vi "cs-scanning_ssxy.vi"() -> ()   [LabVIEW 2017]
uses:
  controls/boolean_info.ctl
  controls/z-axis-params_ssxy.ctl
  <vilib>/rvi/Emulation/niFpgaGetClockAttributes.vi
  <vilib>/rvi/Emulation/niFpgaSctlEmulationGetInTimedLoop.vi
  <vilib>/rvi/Emulation/niFpgaEmulationReportErrorSimple.vi
  <vilib>/rvi/Emulation/niFpgaProcessEmulError.vi
  <vilib>/rvi/eio/common/nirviEmuTemplateMethod_errors.vi
  <vilib>/rvi/Emulation/niFpgaCriticalErrorInLSC.vi
  <vilib>/rvi/Emulation/niFpgaEmulationIsFPGAContextNoSignature.vi
  <vilib>/rvi/DataTransferAndStorage/Container/Common/niFpgaContainerGetUniqueNameForEmu.vi
  <vilib>/rvi/Memory/Memory_Emulation/niFpgaMemoryEmulationCacheClearOnFirstRun.vi
  <vilib>/rvi/Memory/Memory_Emulation/nirvimemoryEmulationManagerCache_MakeExclusive.vi
  <vilib>/rvi/Memory/Memory_Emulation/niFpgaMemoryEmulationValidateCache.vi
  <vilib>/rvi/Memory/Memory_Emulation/nirvimemoryEmulationManagerCache_InsertValue.vi
  <vilib>/Utility/error.llb/Clear Errors.vi
  <vilib>/rvi/Memory/Memory_Emulation/nirvimemoryEmulationManagerCache_ReleaseExclusive.vi
  <vilib>/rvi/Memory/Memory_Emulation/nirvimemoryEmulationManagerCache_GetValue.vi
  <vilib>/rvi/Memory/Memory_Emulation/nirvimemoryEmulationManagerCache_SetValue.vi
  <vilib>/eio/EIONode/EIONode.xnode
  <vilib>/rvi/DataTransferAndStorage/Container/XNode/niFpgaContainer.xnode
  <vilib>/rvi/DataTransferAndStorage/Register/Emulation/niFpgaRegisterEmulation.vi
  FPGA-data-logging.lvlib
  libimaging-cs.lvlib
panel:
  out "xy(k)":fxp<+/-,17,6>[](array[numeric])
  out "ref-data":fxp<+/-,16,5>[](array[numeric])
  out "u_y saturated":bool
  out "u_x saturated":bool
  in  "Ki-xy 2":sgl=0.001 format="%#_13g"
  in  "xy-bound 2":sgl
  out "scaning finished 2":bool
  out "scaning finished":bool
  out "Stopped 2":bool
  in  "z_axis_params":T1={"TOL"=0.29998779296875, "ramp_rate"=-5e-06, "z_u_max"=5.0, "setpoint"=0.0, "Ki"=0.001007080078125, "Z_error_threshold"=0.0, "Z_settled_samples_threshold "=0, "z_UP"=1.5, "zup_N"=5000} {"Z_error_threshold" format="%#_13g"; "ramp_rate" format="%#_4g"; "TOL" format="%#_13g"}
  in  "Kiz_down":sgl format="%#_13g"
  in  "max_Z_settle_samples":i16
  in  "step_down_frac":fxp<+,8,1>
  in  "collect all":bool
  out "iter":i32
  out "entity-index":i16
  in  "TsTicks":u32=1600
  out "number-settled-samples-Z":i16
  out "State":i8
  out "boolean \nindicators":T2
  out "z-u(k)":fxp<+/-,16,5>
  in  "ABORT":bool
  out "read fifo timeout":bool
  in  "numEntities":i16
  in  "init Z up":fxp<+/-,16,5>
  in  "trigger-0":bool
  out "number-settled-samples-y":i16
  out "number-settled-samples-x":i16
  in  "xy-error-threshold":sgl format="%#_13g"
  in  "settled-samples\nthreshold":i16
  in  "initial case":i8
  # "- If collect all = fasle and collect move = false,\nwe only collect measurement data.\n- If collect all = false, and collect move = true,\nwe collect measurement and move data.\n- If collect all = true, we collect everything."
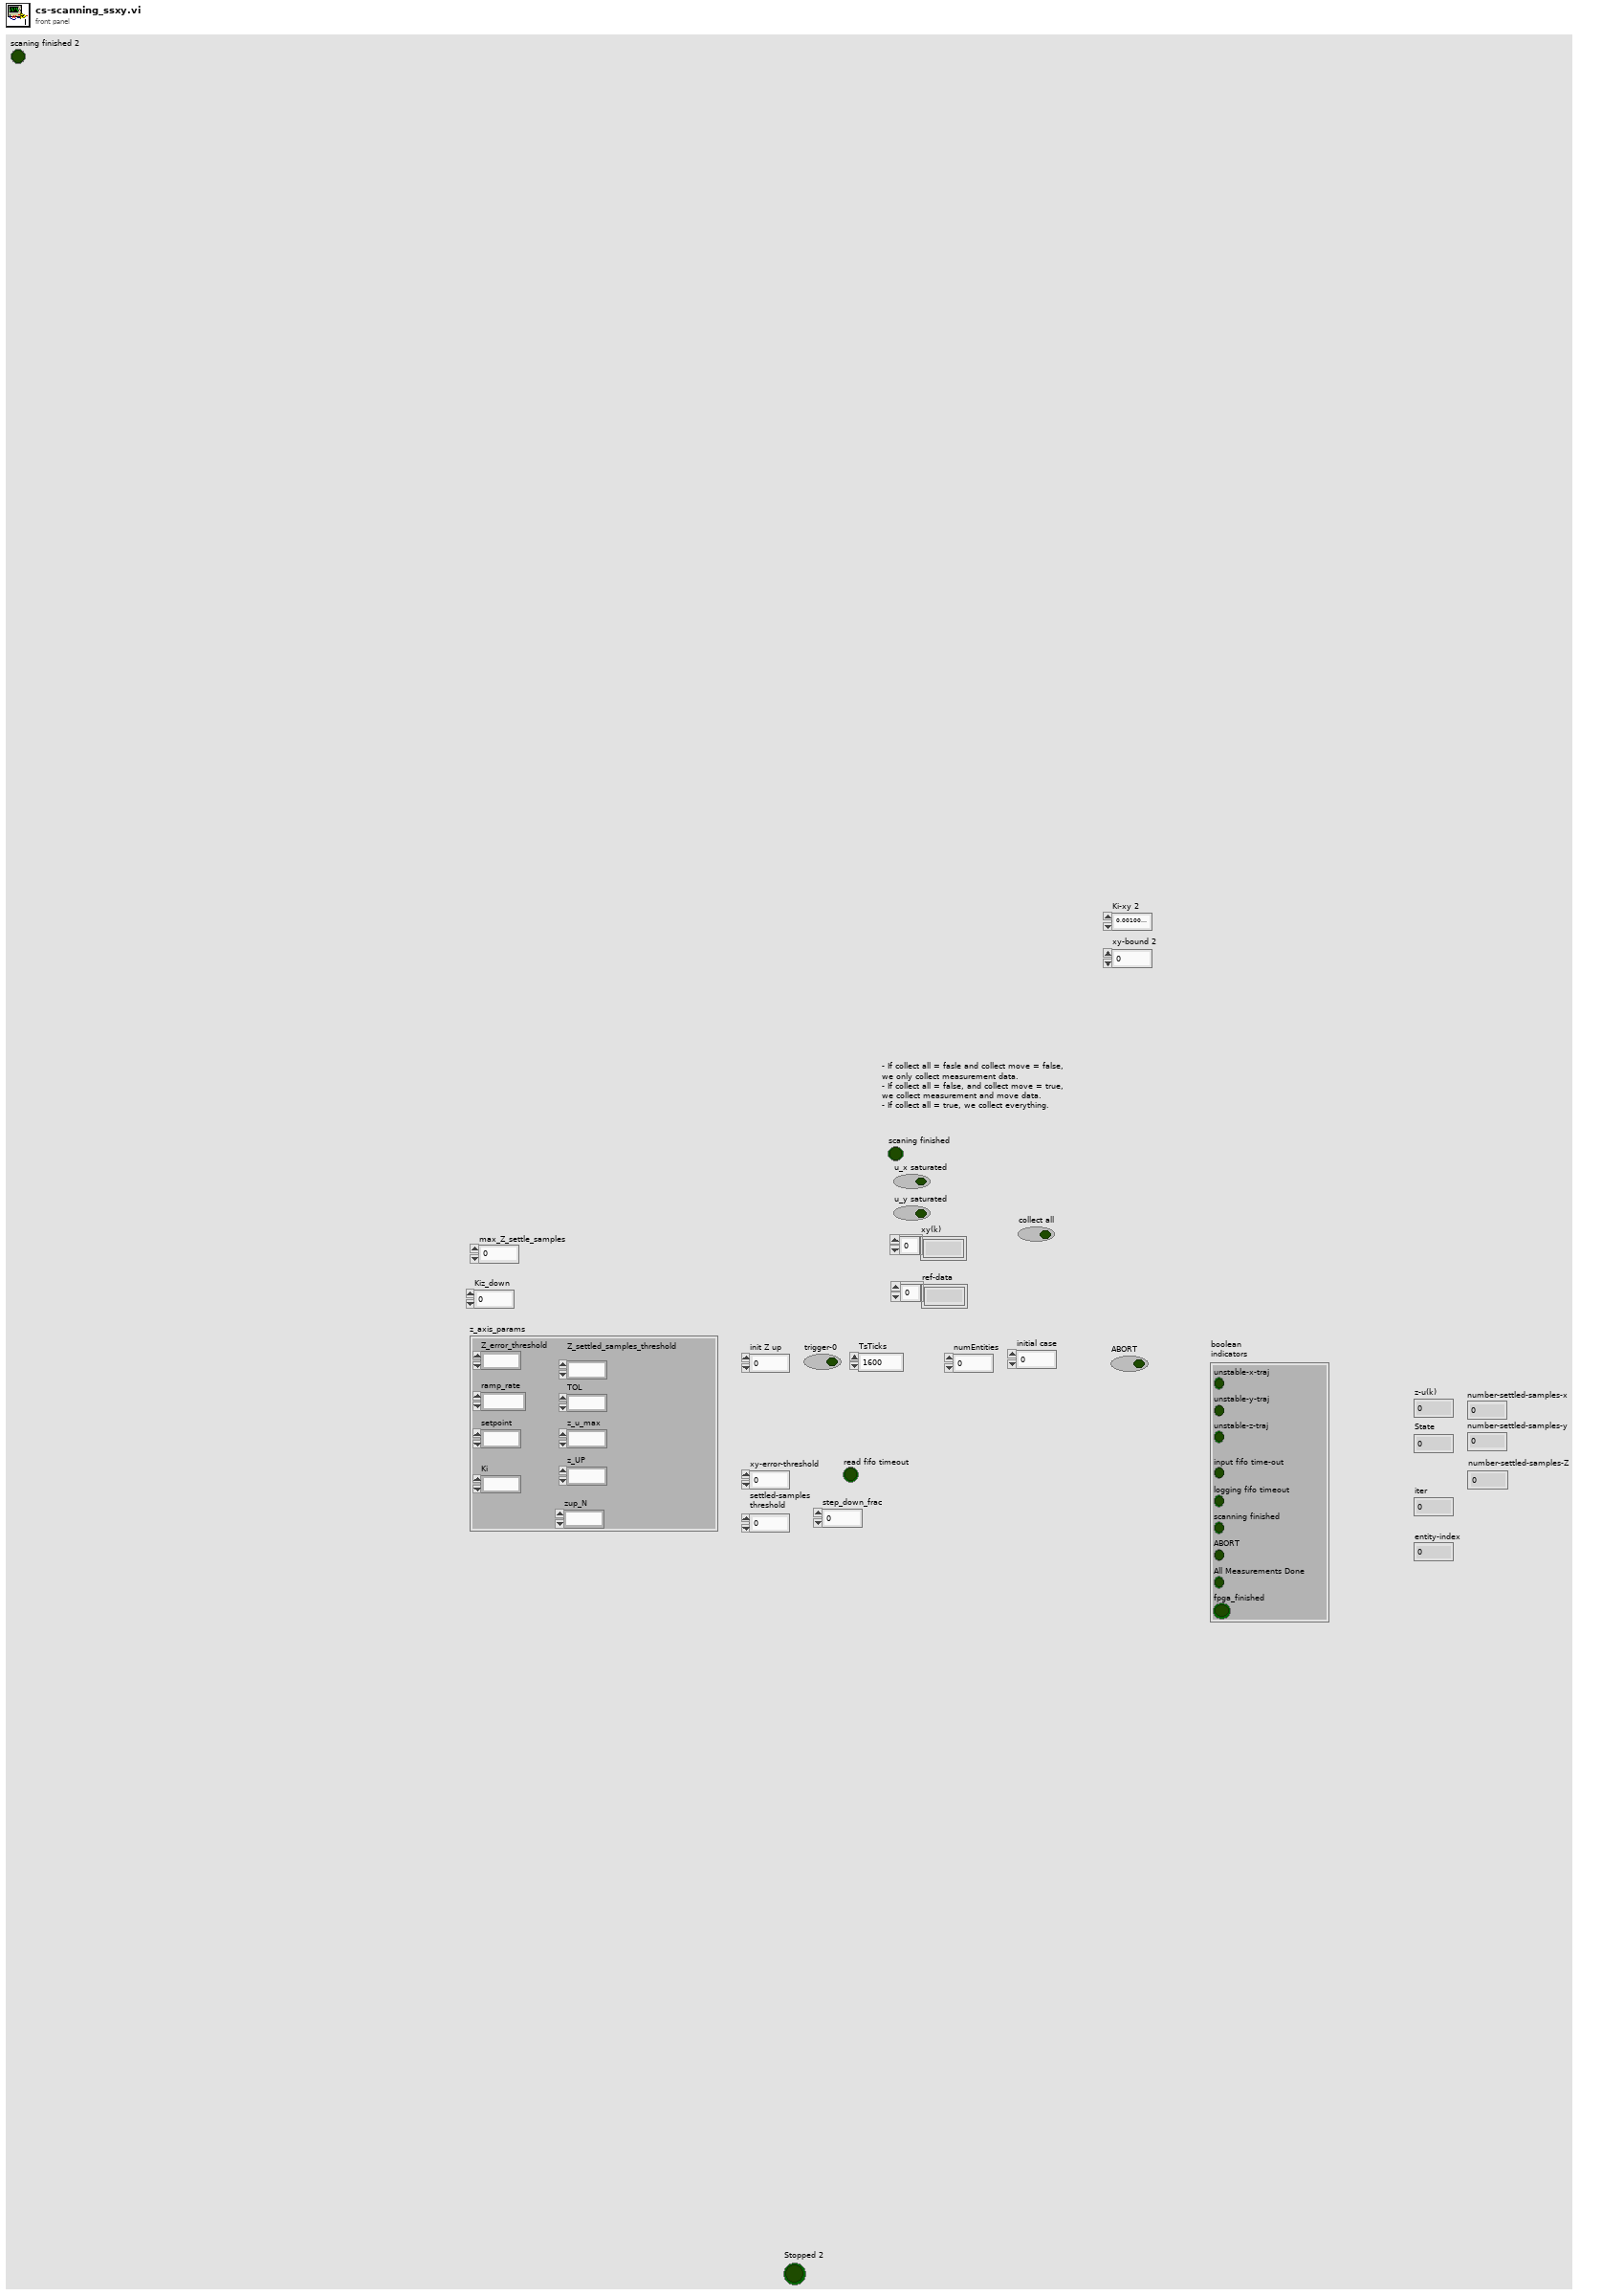
[diagram p1: front panel]
types:
  T1 = typedef "z-axis-params_ssxy.ctl" = cluster{"TOL":fxp<+/-,16,2>, "ramp_rate":sgl, "z_u_max":fxp<+/-,16,5>, "setpoint":fxp<+/-,16,5>, "Ki":fxp<+,16,1>, "Z_error_threshold":fxp<+/-,16,5>, "Z_settled_samples_threshold ":i16, "z_UP":fxp<+/-,16,5>, "zup_N":i16}
  T2 = typedef "boolean_info.ctl" = cluster{"unstable-z-traj":bool, "input fifo time-out":bool, "logging fifo timeout":bool, "scanning finished":bool, "unstable-x-traj":bool, "unstable-y-traj":bool, "ABORT":bool, "All Measurements Done":bool, "fpga_finished":bool}
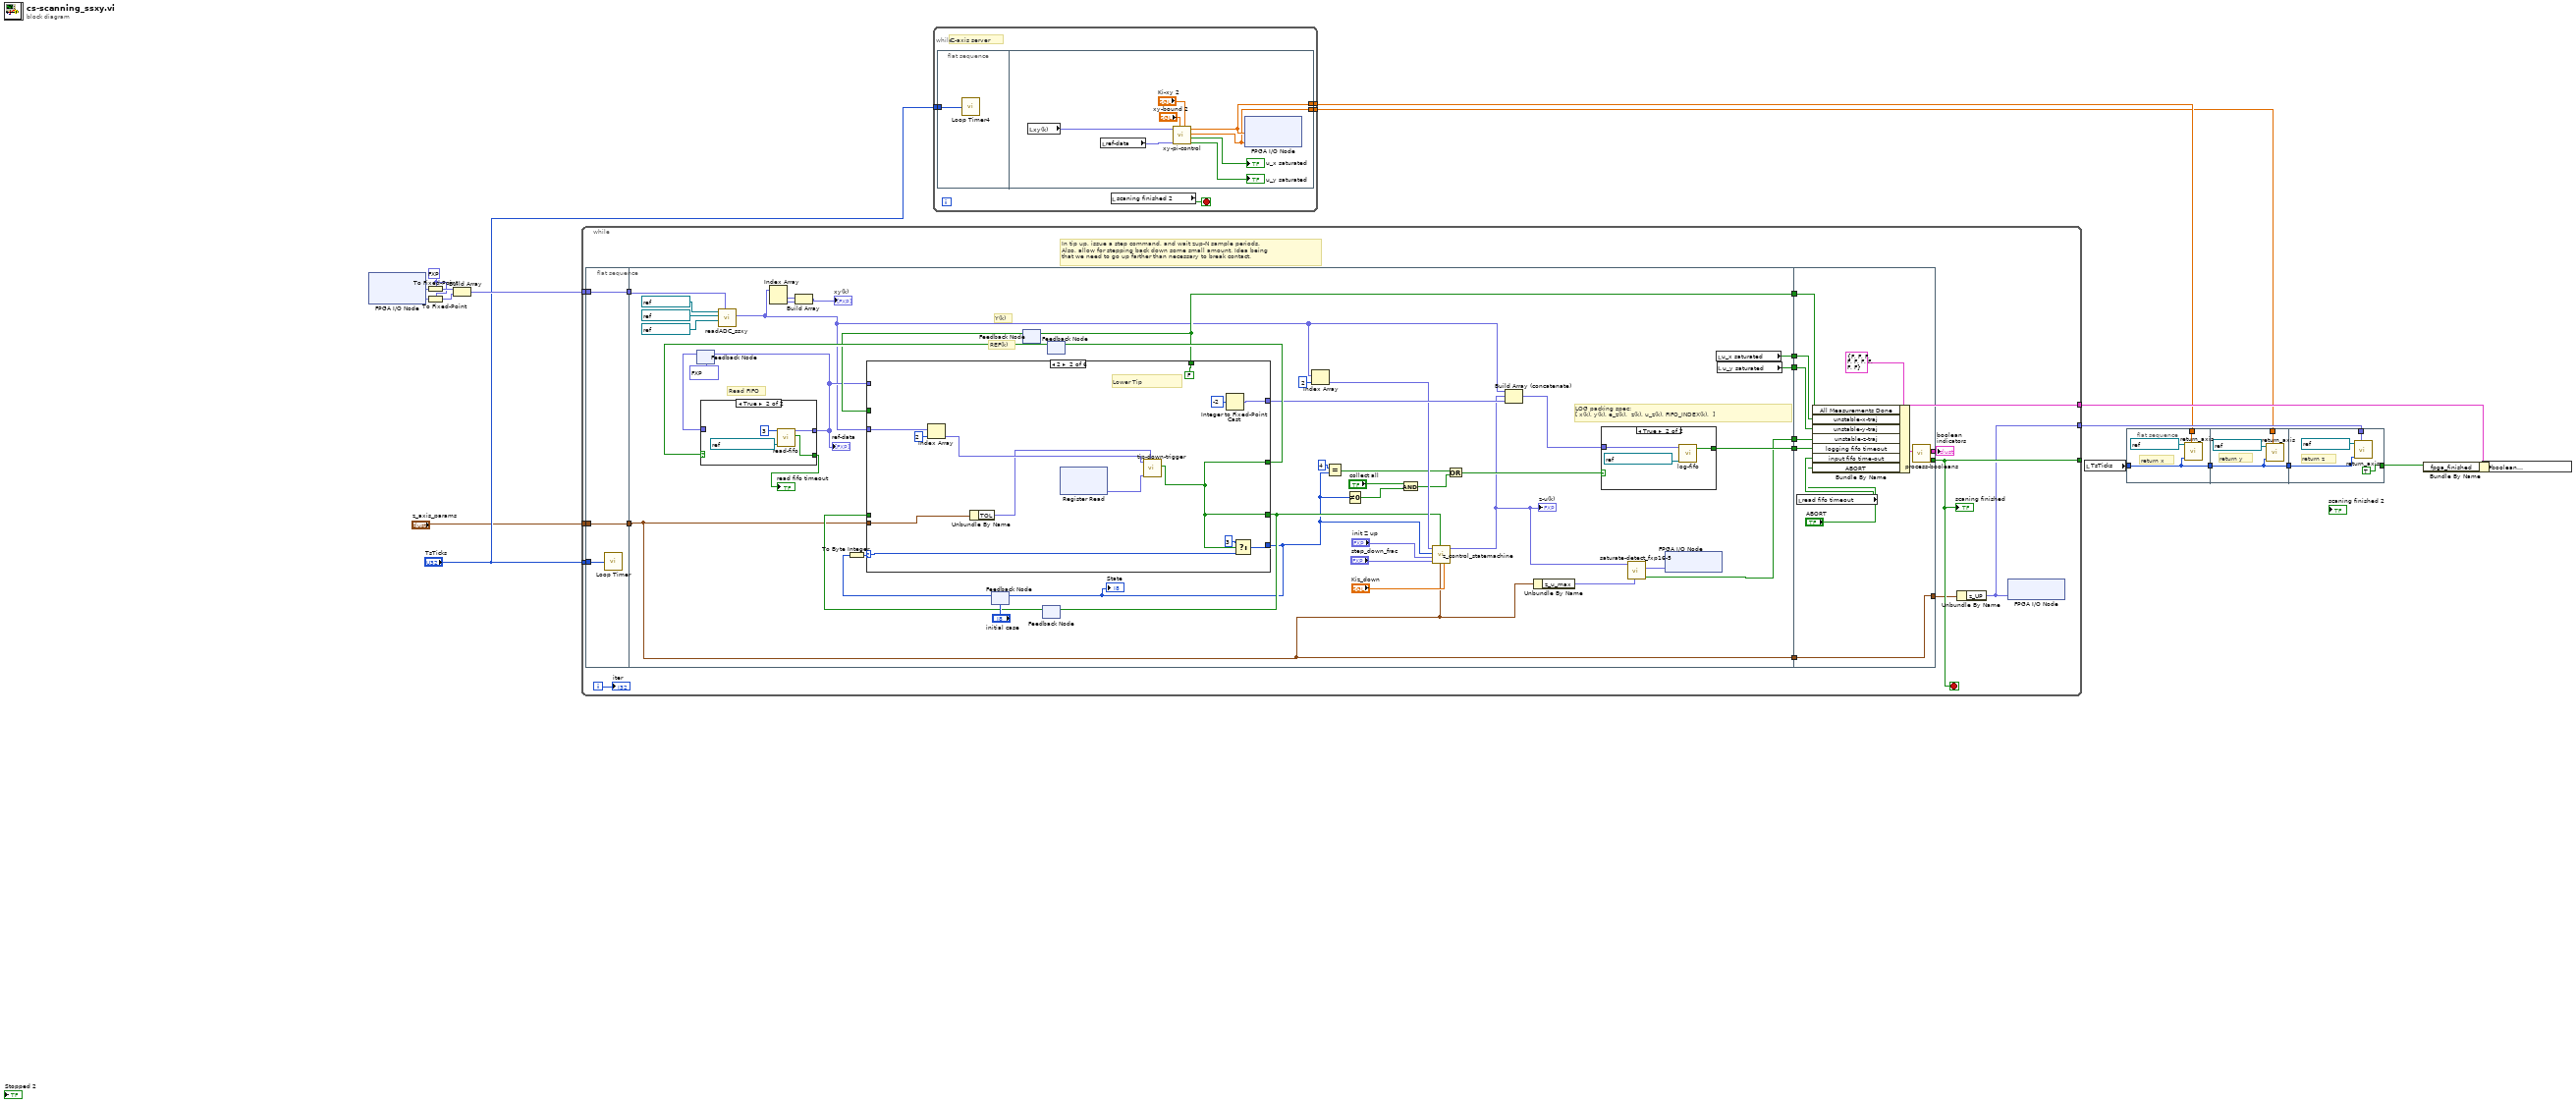
[diagram p0: block diagram]
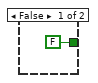
[diagram p2: hidden frame]
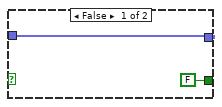
[diagram p3: hidden frame]
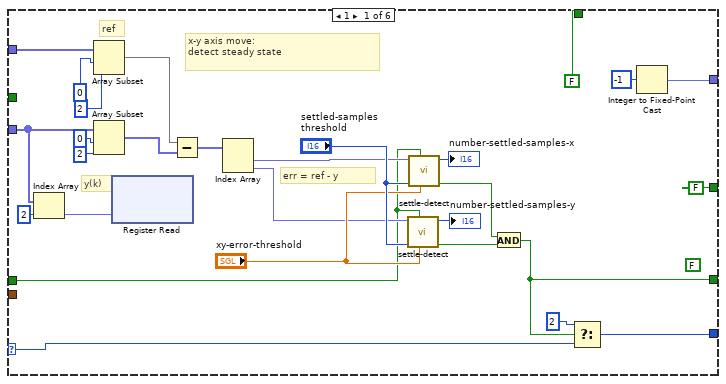
[diagram p4: hidden frame]
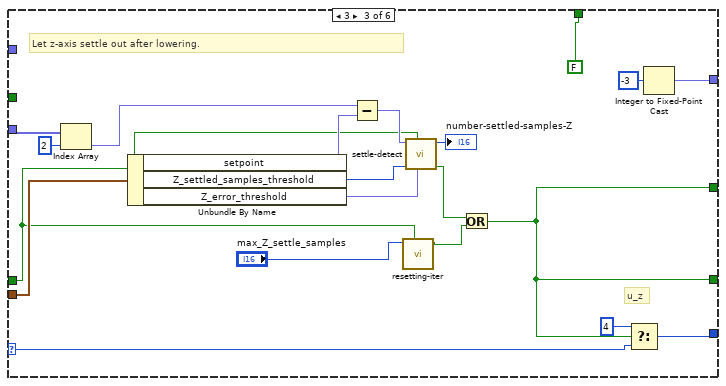
[diagram p5: hidden frame]
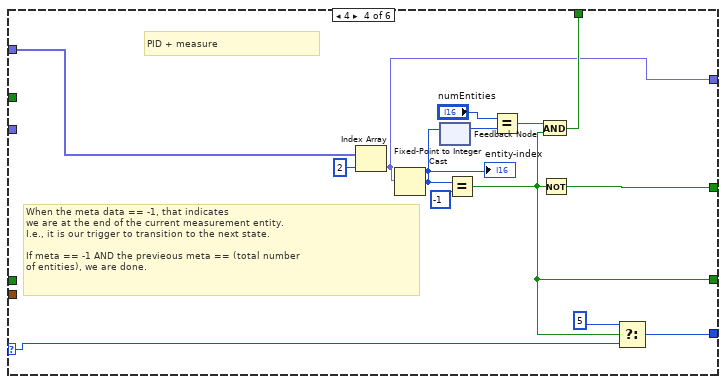
[diagram p6: hidden frame]
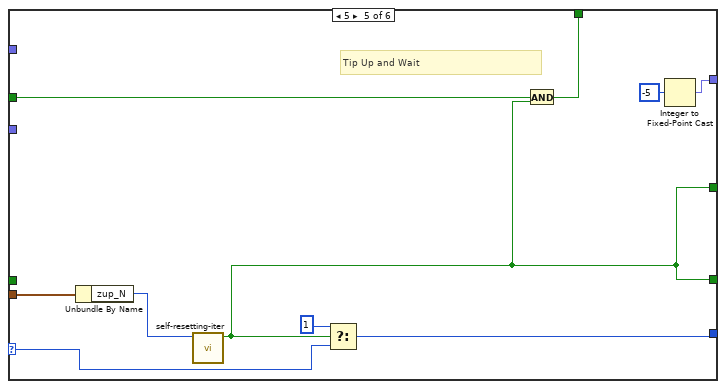
[diagram p7: hidden frame]
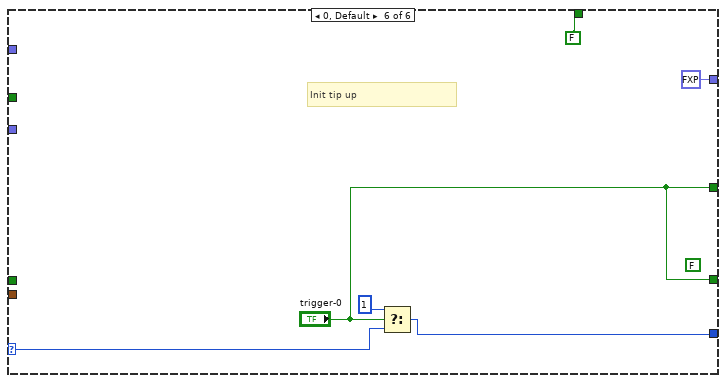
[diagram p8: hidden frame]
diagram:
  w12 = fxp<+/-,16,5> 0.0 ("fixed-point type")
  n1 = xnode "FPGA I/O Node"() -> ("Mod2/AI0"=w15:fxp<+/-,24,5>, "Mod2/AI1"=w13:fxp<+/-,24,5>)  [unwired: 2 in, 2 out]
  n2 = To Fixed-Point(fixed-point type=w12, number=w15) -> (fixed-point=w17:fxp<+/-,16,5>)
  n3 = To Fixed-Point(fixed-point type=w12, number=w13) -> (fixed-point=w14:fxp<+/-,16,5>)
  n4 = Build Array(w17, w14) -> (w16:fxp<+/-,16,5>[])
  n5 = while {
    tunnel: w16 -> [w26]
    tunnel: "z_axis_params" -> [w25]
    tunnel: "TsTicks" -> [w24]
    tunnel: [w23] -> _
    tunnel: [w21] -> w8
    tunnel: [w18] -> w5
    i -> [w22]
    stop <- w23 stop-if-true
    # "In tip up, issue a step command, and wait zup-N sample periods.\nAlso, allow for stepping back down some small amount. Idea being \nthat we need to go up farther than necessary to break contact."
    n6 = flat-sequence {
      tunnel: w26 -> [w36]
      tunnel: [w36] -> w33
      tunnel: w24 -> [w34]
      tunnel: w25 -> [w35]
      tunnel: [w35] -> w32
      tunnel: w33 -> [w64]
      tunnel: w32 -> [w41]
      tunnel: [w58] -> w31
      tunnel: [w57] -> w30
      tunnel: [w42] -> w29
      tunnel: [w76] -> w28
      tunnel: [w66] -> w27
      tunnel: [w41] -> w20
      tunnel: w31 -> [w192]
      tunnel: w30 -> [w191]
      tunnel: w29 -> [w190]
      tunnel: w28 -> [w187]
      tunnel: w27 -> [w184]
      tunnel: [w183] -> w23
      tunnel: [w182] -> w21
      tunnel: w20 -> [w181]
      tunnel: [w181] -> w19
      frame #0 {
        n7 = call "Loop Timer"("Count(Ticks)"=w34) -> ()  [unwired: 1 out]
      }
      frame #1 {
        # "REF(k)"
        # "Y(k)"
        # "LOG packing spec:\n[ x(k), y(k), e_z(k),  z(k), u_z(k), FIFO_INDEX(k),  ]"
        # "Read FIFO"
        n8 = feedback #1(fxp<+/-,16,5>[] [0.0, 0.0, 0.0] ("unpacked-data")) -> (w78:fxp<+/-,16,5>[])
        n9 = call "readADC_ssxy.vi"("x(0), y(0)"=w64, "z-err- ADC"=refnum<k21> "Mod2/AI2" ("y - ADC"), "y - ADC"=refnum<k21> "Mod2/AI1", "x - ADC"=refnum<k21> "Mod2/AI0") -> ("x_y_ze_z_k"=w40:fxp<+/-,17,6>[])  [unwired: 7 in]
        n10 = Index Array(array=w40) -> (element #1=w39:fxp<+/-,17,6>, element #2=w38:fxp<+/-,17,6>)  [unwired: 2 in]
        n11 = Build Array(w39, w38) -> (→"xy(k)":fxp<+/-,17,6>[])
        n12 = feedback #2("initial case") -> (w59:i8)
        n13 = To Byte Integer(number=w59) -> (8bit integer=w60:i8)
        n14 = feedback #3() -> (w71:bool)  [unwired: 1 in]
        n15 = feedback #4() -> (w70:bool)  [unwired: 1 in]
        n16 = feedback #5() -> (w73:bool)  [unwired: 1 in]
        n17 = case shown="True" w73 {
          tunnel: w78 -> [w85 _]
          tunnel: [w85 w87] -> w56
          tunnel: [FALSE ("timout?") w86] -> w75
          frame False {
          }
          frame True {
            n18 = call "read-fifo.vi"("FIFO In"=refnum<k21> "Host_to_FPGA", "numChan"=3) -> ("timout?"=w86:bool, "unpacked-data"=w87:fxp<+/-,16,5>[])  [unwired: 8 in]
          }
        }
        "read fifo timeout" <- w75
        "ref-data" <- w56
        n19 = feedback-in #1(w56) -> ()
        n20 = case shown="2" w60 {
          selector: w60 -> [w109 w130 w143 w162 w174 w178]
          tunnel: [w110 w125 w144 w163 w173 w180] -> w47
          tunnel: w40 -> [w91 w127 w148 _ _ _]
          tunnel: [FALSE w120 w134 w155 w167 "trigger-0"] -> w74
          tunnel: w41 -> [_ w129 w142 _ w171 _]
          tunnel: [FALSE FALSE FALSE w154 w165 FALSE] -> w66
          tunnel: w71 -> [_ _ _ _ w169 _]
          tunnel: w70 -> [w99 _ w131 _ _ _]
          tunnel: [w97 w120 w134 w153 w167 "trigger-0"] -> w52
          tunnel: [w94 w121 w137 w152 w166 fxp<+/-,16,5> 0.0 ("Element")] -> w67
          tunnel: w56 -> [w90 _ _ w151 _ _]
          frame 1 {
            (unwired) FALSE ("trigger-0")
            # "y(k)"
            # "err = ref - y"
            # "ref"
            # "x-y axis move: \ndetect steady state"
            n21 = Index Array(array=w91, index=2) -> (element=w93:fxp<+/-,17,6>)
            n22 = Array Subset(array=w90, index=0, length=2) -> (w104:fxp<+/-,16,5>[])
            n23 = Array Subset(array=w91, index=0, length=2) -> (w103:fxp<+/-,17,6>[])
            n24 = xnode ("Register Read")("Data"=w93) -> ()  [unwired: 1 in, 1 out]
            n25 = Subtract(x=w104, y=w103) -> (x-y=w96:fxp<+/-,18,7>[])
            n26 = Index Array(array=w96) -> (element #1=w102:fxp<+/-,18,7>, element #2=w101:fxp<+/-,18,7>)  [unwired: 2 in]
            n27 = call "settle-detect.vi"("error-max"="xy-error-threshold", "reset"=w99, "settled-samples\nthreshold"="settled-samples\nthreshold", "err(k)"=w101) -> ("has-settled"=w117:bool, "number-settled-samples"=→"number-settled-samples-y":u16)  [unwired: 6 in]
            n28 = call "settle-detect.vi"("error-max"="xy-error-threshold", "reset"=w99, "settled-samples\nthreshold"="settled-samples\nthreshold", "err(k)"=w102) -> ("has-settled"=w116:bool, "number-settled-samples"=→"number-settled-samples-x":u16)  [unwired: 6 in]
            n29 = And(x=w116, y=w117) -> (x .and. y?=w97:bool)
            n30 = Select(t=i8 2, s=w97, f=w109) -> (s? t:f=w110:i8)
            n31 = Integer to Fixed-Point Cast(integer=i16 -1) -> (fixed-point=w94:fxp<+/-,16,5>)  [unwired: 1 in]
          }
          frame 2 {
            # "Lower Tip"
            n32 = Index Array(array=w127, index=2) -> (element=w126:fxp<+/-,17,6>)
            n33 = Unbundle By Name(w129) -> ("TOL"=w119:fxp<+/-,16,2>)
            n34 = xnode ("Register Read")() -> ("Data"=w118:fxp<+/-,16,5>)  [unwired: 1 in, 1 out]
            n35 = call "tip-down-trigger.vi"("TOL"=w119, "Vo"=w118, "e(k)"=w126) -> ("trigger"=w120:bool)  [unwired: 8 in]
            n36 = Integer to Fixed-Point Cast(integer=i16 -2) -> (fixed-point=w121:fxp<+/-,16,5>)  [unwired: 1 in]
            n37 = Select(t=i8 3, s=w120, f=w130) -> (s? t:f=w125:i8)
          }
          frame 3 {
            # "u_z"
            # "Let z-axis settle out after lowering."
            n38 = Index Array(array=w148, index=2) -> (element=w146:fxp<+/-,17,6>)
            n39 = Unbundle By Name(w142) -> ("setpoint"=w136:fxp<+/-,16,5>, "Z_settled_samples_threshold"=w141:i16, "Z_error_threshold"=w140:fxp<+/-,16,5>)
            n40 = Subtract(x=w146, y=w136) -> (x-y=w149:fxp<+/-,18,7>)
            n41 = call "resetting-iter.vi"("reset"=w131, "N"="max_Z_settle_samples") -> ("Boolean"=w133:bool)  [unwired: 8 in, 1 out]
            n42 = call "settle-detect.vi"("error-max"=w140, "reset"=w131, "settled-samples\nthreshold"=w141, "err(k)"=w149) -> ("has-settled"=w135:bool, "number-settled-samples"=→"number-settled-samples-Z":u16)  [unwired: 6 in]
            n43 = Or(x=w135, y=w133) -> (x .or. y?=w134:bool)
            n44 = Select(t=i8 4, s=w134, f=w143) -> (s? t:f=w144:i8)
            n45 = Integer to Fixed-Point Cast(integer=i16 -3) -> (fixed-point=w137:fxp<+/-,16,5>)  [unwired: 1 in]
          }
          frame 4 {
            # "When the meta data == -1, that indicates\nwe are at the end of the current measurement entity.\nI.e., it is our trigger to transition to the next state.\n\nIf meta == -1 AND the previeous meta == (total number\nof entities), we are done."
            # "PID + measure"
            n46 = Index Array(array=w151, index=2) -> (element=w152:fxp<+/-,16,5>)
            n47 = Fixed-Point to Integer Cast(1:w152) -> (0:w156:i16)
            "entity-index" <- w156
            n48 = feedback #6() -> (w157:i16)  [unwired: 1 in]
            n49 = feedback-in #6(w156) -> ()
            n50 = Equal?(x=w156, y=i16 -1) -> (x = y?=w153:bool)
            n51 = Equal?(x="numEntities", y=w157) -> (x = y?=w158:bool)
            n52 = And(x=w158, y=w153) -> (x .and. y?=w154:bool)
            n53 = Not(x=w153) -> (.not. x?=w155:bool)
            n54 = Select(t=i8 5, s=w153, f=w162) -> (s? t:f=w163:i8)
          }
          frame 5 {
            # "Tip Up and Wait"
            n55 = Unbundle By Name(w171) -> ("zup_N"=w170:i16)
            n56 = call "self-resetting-iter.vi"("N"=w170) -> ("Boolean"=w167:bool)  [unwired: 9 in, 1 out]
            n57 = Select(t=i8 1, s=w167, f=w174) -> (s? t:f=w173:i8)
            n58 = And(x=w169, y=w167) -> (x .and. y?=w165:bool)
            n59 = Integer to Fixed-Point Cast(integer=i16 -5) -> (fixed-point=w166:fxp<+/-,16,5>)  [unwired: 1 in]
          }
          frame 0, Default {
            (unwired) FALSE ("trigger-0")
            # "Init tip up"
            n60 = Select(t=i8 1, s="trigger-0", f=w178) -> (s? t:f=w180:i8)
          }
        }
        "State" <- w47
        n61 = feedback-in #2(w47) -> ()
        n62 = feedback-in #3(w66) -> ()
        n63 = feedback-in #4(w52) -> ()
        n64 = feedback-in #5(w74) -> ()
        n65 = Index Array(array=w40, index=2) -> (element=w55:fxp<+/-,17,6>)
        n66 = Equal?(x=i8 4, y=w47) -> (x = y?=w48:bool)
        n67 = Not Equal To 0?(x=w47) -> (x != 0?=w69:bool)
        n68 = And(x="collect all", y=w69) -> (x .and. y?=w50:bool)
        n69 = call "z_control_statemachine.vi"("Kiz_down"="Kiz_down", "z_axis_params"=w41, "step_down"=w52, "step_down_frac"="step_down_frac", "init Z up"="init Z up", "State"=w47, "zerr(k)"=w55) -> ("z-u(k)"=w43:fxp<+/-,16,5>)  [unwired: 4 in]
        "z-u(k)" <- w43
        n70 = Or(x=w48, y=w50) -> (x .or. y?=w49:bool)
        n71 = Build Array (concatenate)(w40, w43, w67) -> (w77:fxp<+/-,17,6>[])
        n72 = Unbundle By Name(w41) -> ("z_u_max"=w44:fxp<+/-,16,5>)
        n73 = case shown="True" w49 {
          tunnel: w77 -> [_ w82]
          tunnel: [FALSE ("logging-timeout?") w81] -> w76
          frame False {
          }
          frame True {
            n74 = call "log-fifo.vi"("FIFO In"=refnum<k21> "fpga-to-host2", "input-data"=w82) -> ("logging-timeout?"=w81:bool)  [unwired: 9 in]
          }
        }
        n75 = call "saturate-detect_fxp16-5.vi"("bound"=w44, "x"=w43) -> ("saturated"=w42:bool, "sat(x)"=w45:fxp<+/-,16,5>)  [unwired: 8 in]
        n76 = xnode "FPGA I/O Node"("Mod1/AO2"=w45) -> ()  [unwired: 1 in, 1 out]
        n77 = local read "u_x saturated"() -> (w58:bool)
        n78 = local read "u_y saturated"() -> (w57:bool)
      }
      frame #2 {
        n79 = local read "read fifo timeout"() -> (w186:bool)
        n80 = Bundle By Name(cluster=T2 {"unstable-z-traj"=FALSE, "input fifo time-out"=FALSE, "logging fifo timeout"=FALSE, "scanning finished"=FALSE, "unstable-x-traj"=FALSE, "unstable-y-traj"=FALSE, "ABORT"=FALSE, "All Measurements Done"=FALSE, "fpga_finished"=FALSE} ("boolean errors"), "All Measurements Done"=w184, "unstable-x-traj"=w192, "unstable-y-traj"=w191, "unstable-z-traj"=w190, "logging fifo timeout"=w187, "input fifo time-out"=w186, "ABORT"="ABORT") -> (w188:T2)
        n81 = call "process-booleans.vi"("boolean indicators 2"=w188) -> ("scaning finished"=w183:bool, "boolean indicators"=w182:T2)  [unwired: 9 in]
      }
    }
    n82 = Unbundle By Name(w19) -> ("z_UP"=w18:fxp<+/-,16,5>)
    n83 = xnode "FPGA I/O Node"("Mod1/AO2"=w18) -> ()  [unwired: 1 in, 1 out]
    "boolean \nindicators" <- w21
    "iter" <- w22
    "scaning finished" <- w23
  }
  n84 = while {
    tunnel: "TsTicks" -> [w196]
    tunnel: [w194] -> w3
    tunnel: [w193] -> w2
    stop <- w195 stop-if-true
    # "Z-axis server"
    n85 = flat-sequence {
      tunnel: w196 -> [w197]
      tunnel: [w201] -> w194
      tunnel: [w200] -> w193
      frame #0 {
        n86 = call "Loop Timer4"("Count(Ticks)"=w197) -> ()  [unwired: 1 out]
      }
      frame #1 {
        n87 = local read "xy(k)"() -> (w198:fxp<+/-,17,6>[])
        n88 = local read "ref-data"() -> (w199:fxp<+/-,16,5>[])
        n89 = call "xy-pi-control.vi"("Ki-xy"="Ki-xy 2", "xy-umax"="xy-bound 2", "xy-ref"=w199, "x_k-y_k"=w198) -> ("u_y saturated"=→"u_y saturated":bool, "u_x saturated"=→"u_x saturated":bool, "sat(u_y)"=w200:sgl, "sat(u_x)"=w201:sgl)  [unwired: 4 in]
        n90 = xnode "FPGA I/O Node"("Mod1/AO0"=w201, "Mod1/AO1"=w200) -> ()  [unwired: 2 in, 2 out]
      }
    }
    n91 = local read "scaning finished 2"() -> (w195:bool)
  }
  n92 = local read "TsTicks"() -> (w9:u32)
  n93 = flat-sequence {
    tunnel: w9 -> [w207]
    tunnel: w3 -> [w208]
    tunnel: [w207] -> w11
    tunnel: w2 -> [w211]
    tunnel: w11 -> [w209]
    tunnel: [w209] -> w10
    tunnel: w5 -> [w215]
    tunnel: w10 -> [w213]
    tunnel: [TRUE] -> w7
    frame #0 {
      # "return x"
      n94 = call "return_axis.vi"("u(0)"=w208, "TsTicks"=w207, "FPGA I/O In"=refnum<k21> "Mod1/AO0") -> ()  [unwired: 9 in]
    }
    frame #1 {
      # "return y"
      n95 = call "return_axis.vi"("u(0)"=w211, "TsTicks"=w209, "FPGA I/O In"=refnum<k21> "Mod1/AO1") -> ()  [unwired: 9 in]
    }
    frame #2 {
      # "return z"
      n96 = call "return_axis.vi"("u(0)"=w215, "TsTicks"=w213, "FPGA I/O In"=refnum<k21> "Mod1/AO2") -> ()  [unwired: 9 in]
    }
  }
  n97 = Bundle By Name(cluster=w8, "fpga_finished"=w7) -> (w6:T2)
  n98 = local write "boolean \nindicators"(w6) -> ()
